vi "smart_home.vi"() -> ()   [LabVIEW 2023]
panel:
  in  "?":string
  in  "?":string
  in  "?":string
  out "Gas":bool
  in  "Relay":bool
  in  "?":bool
  out "Motion":bool
  out "Air pressure":dbl
  out "Thermometer":dbl(slide) scale=0.0..50.0
  out "Time":string
  out "Date":string
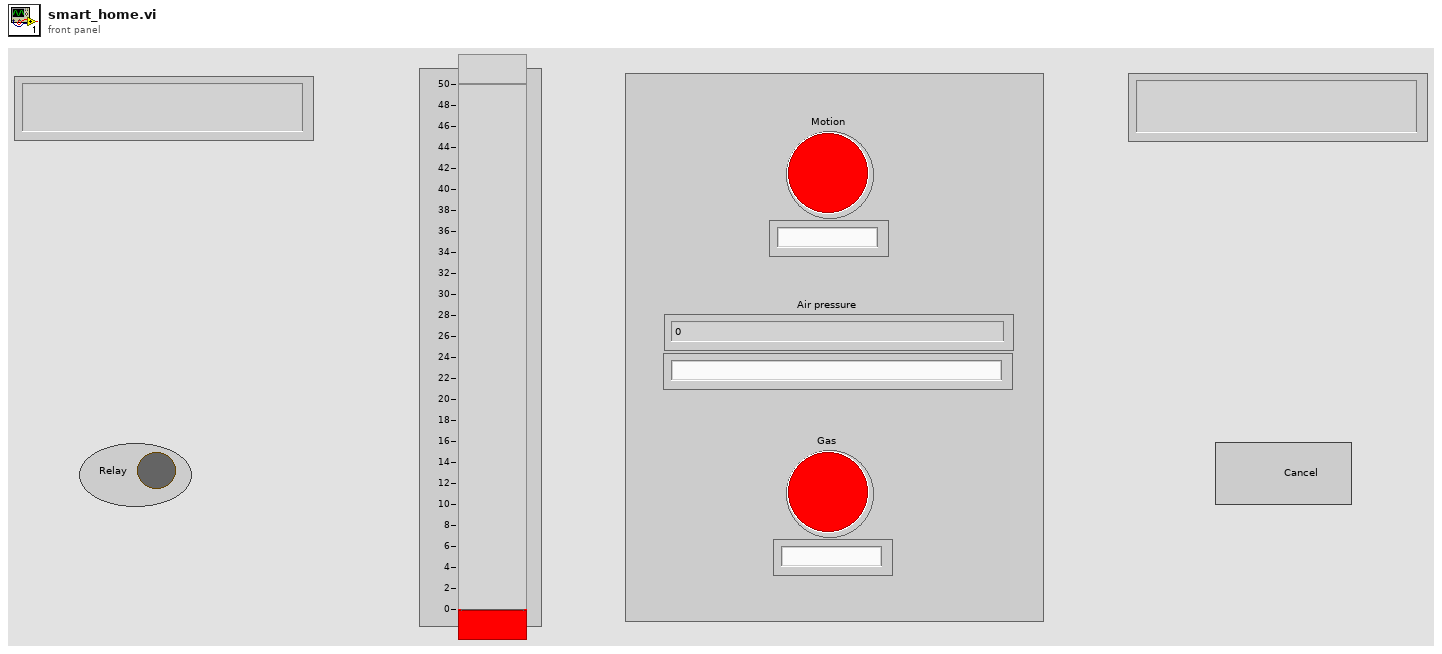
[diagram p1: front panel]
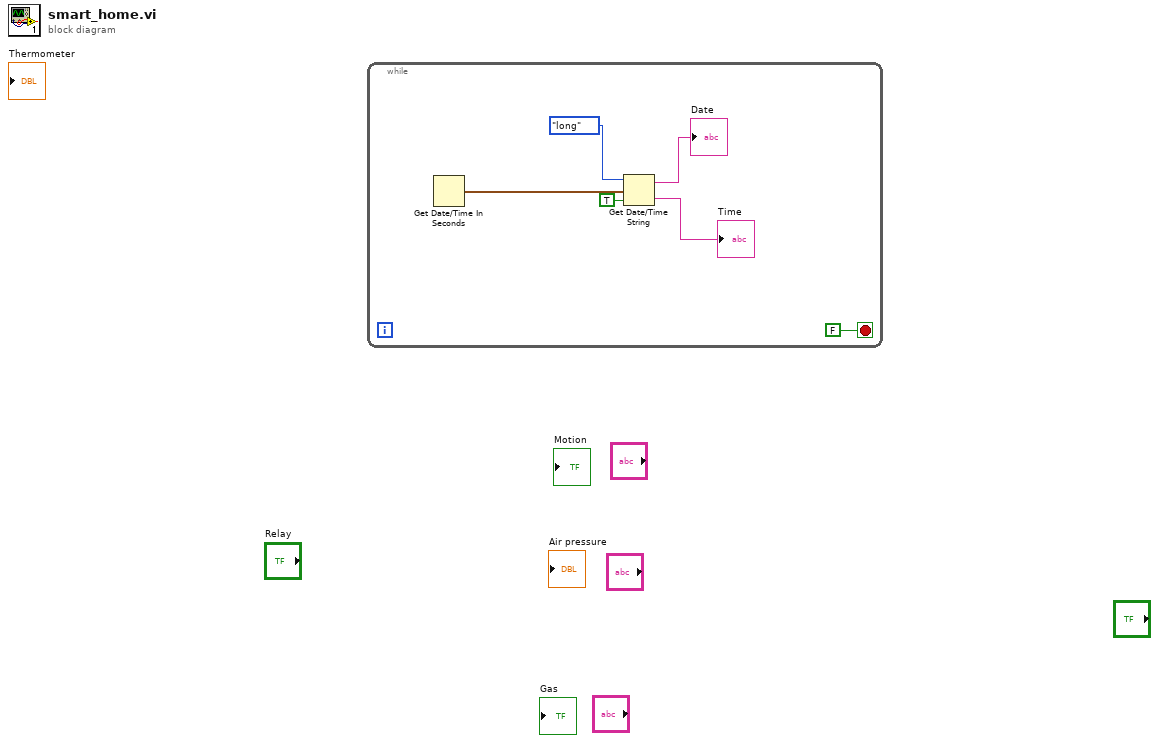
[diagram p0: block diagram]
diagram:
  n1 = while {
    stop <- FALSE stop-if-true
    n2 = Get Date/Time In Seconds() -> (seconds since 1Jan1904=w6:timestamp)
    n3 = Get Date/Time String(date format (0)=enum16{"short", "long", "abbreviated"}."long", seconds (now)=w6, want seconds? (F)=TRUE) -> (date string=→"Date":string, time string=→"Time":string)
  }
